vi "offset and CV.vi"(11 "volts":sgl[][](array[numeric]) format="%.5f") -> (2 "percent CV":sgl format="%.5f", 3 "mean":sgl format="%.5f")   [LabVIEW 2010]
uses:
  <vilib>/Analysis/NI_AALBase.lvlib
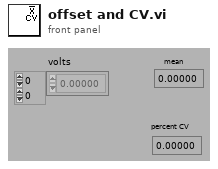
[diagram p1: front panel]
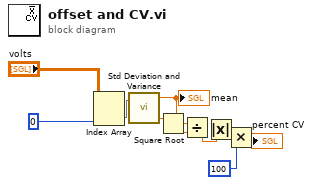
[diagram p0: block diagram]
diagram:
  n1 = Index Array(array="volts", index (col)=0 ("Index")) -> (element=w6:sgl[])  [unwired: 1 in]
  n2 = call <vilib>:"Std Deviation and Variance.vi"("X"=w6) -> ("mean"=w10:dbl, "variance"=w9:dbl)  [unwired: 1 in, 1 out]
  "mean" <- w10
  n3 = Square Root(x=w9) -> (sqrt(x)=w8:dbl)
  n4 = Divide(x=w8, y=w10) -> (x/y=w7:dbl)
  n5 = Absolute Value(x=w7) -> (abs(x)=w3:dbl)
  n6 = Multiply(x=w3, y=100) -> (x*y=→"percent CV":dbl)
